vi "PassObserverTactic_Init.vi"(0 "object in":refnum<class "PassObserverTactic.lvclass">, 5 "error in (no error)":errorcluster) -> (14 "object out":refnum<class "PassObserverTactic.lvclass">, 19 "error out":errorcluster)   [LabVIEW 2020, in "PassObserverTactic.lvclass"]
uses:
  PassObserverTactic.lvclass
  C:/Users/anton/Desktop/RoboIME/IC/SSL_AI/Tactic_class/Tactic.lvclass
  PassObserverTactic.lvclass/PassObserverTactic.ctl
  Tactic_class/Tactic.lvclass
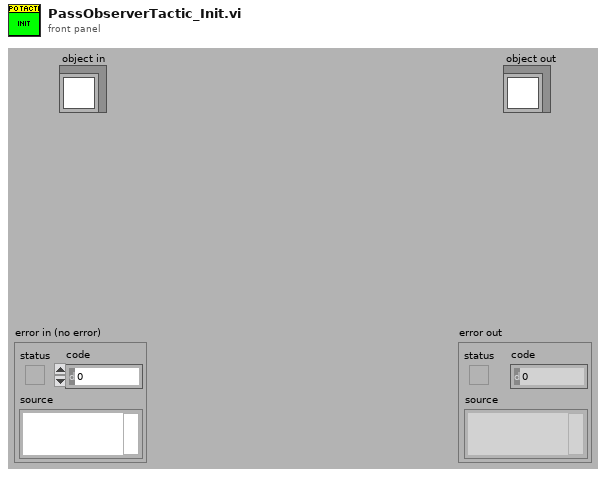
[diagram p1: front panel]
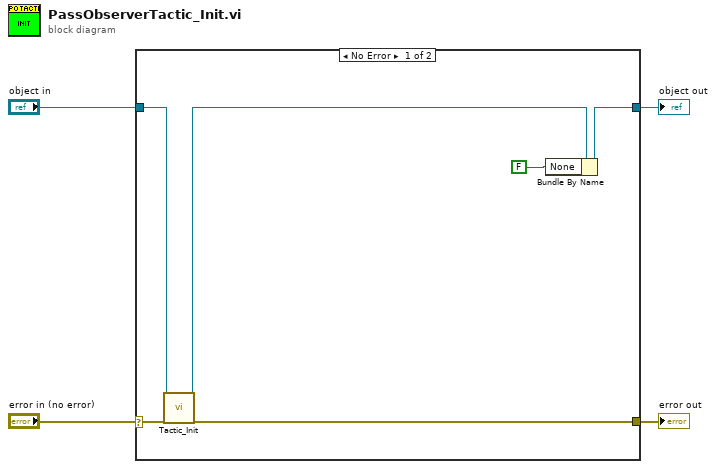
[diagram p0: block diagram]
diagram:
  n1 = case shown="No Error" "error in (no error)" {
    selector: "error in (no error)" -> [w8 w11]
    tunnel: [w10 w12] -> w4
    tunnel: "object in" -> [w6 w12]
    tunnel: [w7 w11] -> w1
    frame No Error {
      n2 = call "Tactic_Init.vi"("object in"=w6, "error in (no error)"=w8) -> ("object out"=w5:refnum<class "PassObserverTactic.lvclass">, "error out"=w7:errorcluster)  [unwired: 16 in]
      n3 = Bundle By Name(cluster=w5, "None"=FALSE) -> (w10:refnum<class "PassObserverTactic.lvclass">)
    }
    frame Error {
    }
  }
  "object out" <- w4
  "error out" <- w1
